vi "Report_Body.vi"(0 "report in":refnum<class "NI_report.lvclass">, 5 "Seq_Measurement":T3(array[cluster]), 7 "General_Info":T1, 9 "Log_Seq":T2(array[cluster]), 11 "error in (no error)":errorcluster) -> (6 "appended path":path, 15 "error out":errorcluster)   [LabVIEW 2023]
uses:
  <vilib>/Utility/NIReport.llb/NI_report.lvclass
  <vilib>/Utility/NIReport.llb/image depth.ctl
  <vilib>/Utility/NIReport.llb/NI_ReportGenerationCore.lvlib
panel:
  out "FFT":cluster{"f0":dbl, "df":dbl, "magnitude":dbl[]}(graph)
  out "Timesignal":waveform(dbl)(graph)
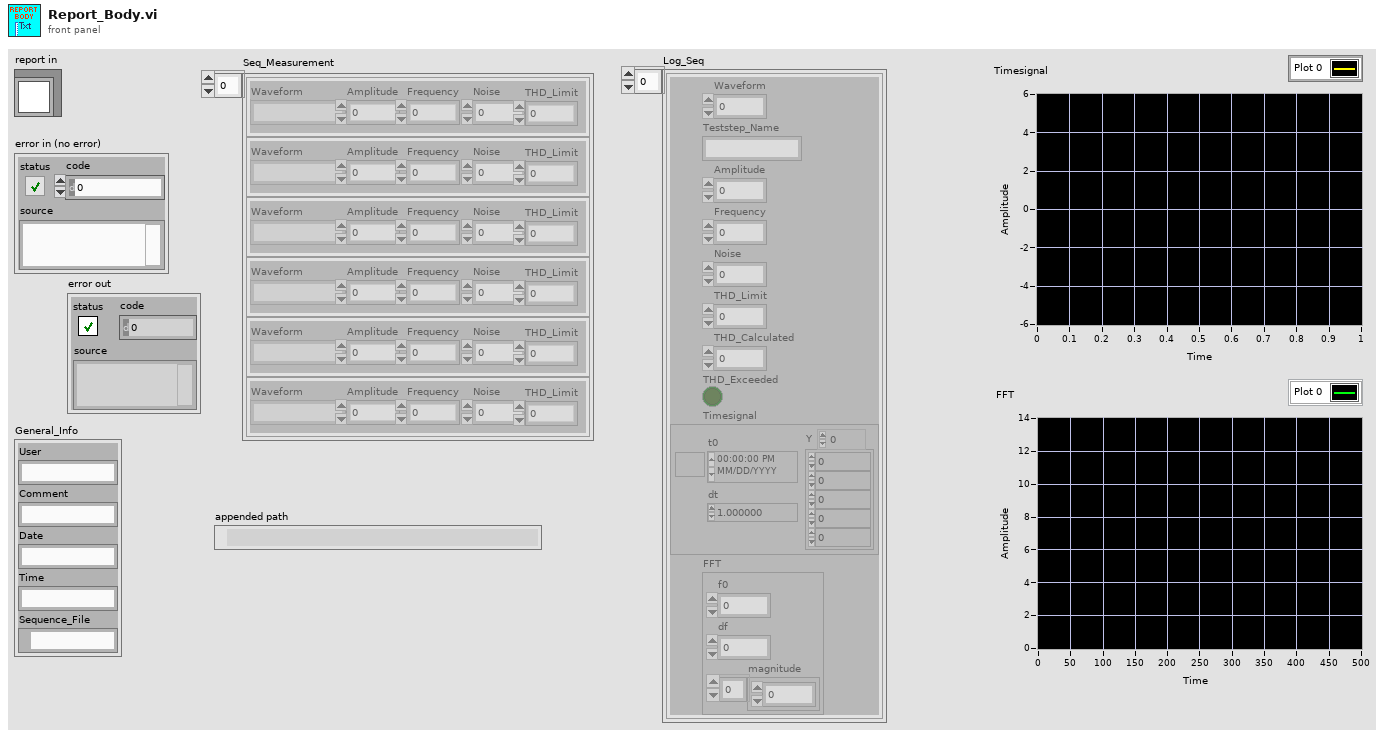
[diagram p1: front panel]
types:
  T1 = cluster{"User":string, "Comment":string, "Date":string, "Time":string, "Sequence_File":path}
  T2 = cluster{"Waveform":i32, "Teststep_Name":string, "Amplitude":dbl, "Frequency":dbl, "Noise":dbl, "THD_Limit":dbl, "THD_Calculated":dbl, "THD_Exceeded":bool, "Timesignal":waveform(dbl), "FFT":cluster{"f0":dbl, "df":dbl, "magnitude":dbl[]}}[]
  T3 = cluster{"Waveform":enum16{"", "Sine Wave", "Triangle Wave", "Square Wave", "Sawtooth Wave"}, "Amplitude":dbl, "Frequency":dbl, "Noise":dbl, "THD_Limit":dbl, "Teststep_Name":string}[]
  T4 = enum16{"open", "replace", "create", "open or create", "replace or create", "replace or create with confirmation"}
  T5 = typedef "NI_ReportGenerationCore.lvlib/image depth.ctl" = u16
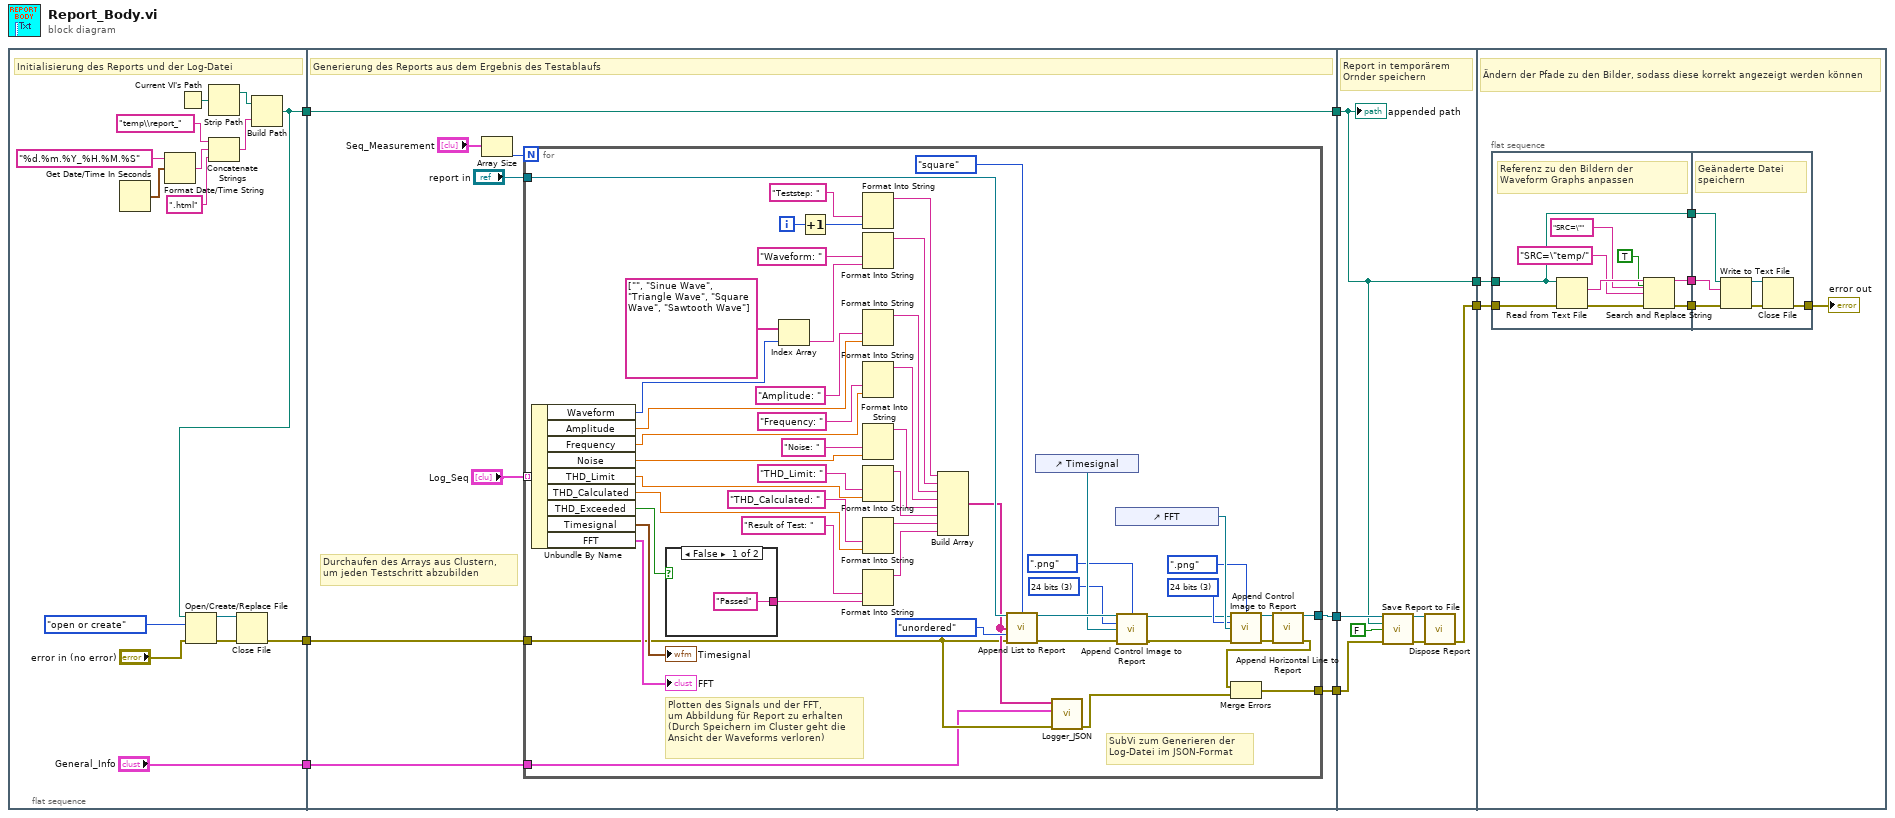
[diagram p0: block diagram]
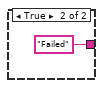
[diagram p2: hidden frame]
diagram:
  n1 = flat-sequence {
    tunnel: [w18] -> w8
    tunnel: [w10] -> w5
    tunnel: ["General_Info"] -> w3
    tunnel: w8 -> [w28]
    tunnel: [w28] -> w7
    tunnel: [w27] -> w6
    tunnel: w5 -> [w26]
    tunnel: [w25] -> w4
    tunnel: w3 -> [w24]
    tunnel: w7 -> [w89]
    tunnel: w6 -> [w93]
    tunnel: w4 -> [w92]
    tunnel: [w89] -> w2
    tunnel: [w88] -> w1
    tunnel: w2 -> [w99]
    tunnel: w1 -> [w98]
    frame #0 {
      # "Initialisierung des Reports und der Log-Datei"
      n2 = Get Date/Time In Seconds() -> (seconds since 1Jan1904=w17:timestamp)
      n3 = Format Date/Time String(time format string (%c)="%d.%m.%Y_%H.%M.%S", seconds (now)=w17) -> (date/time string=w14:string)  [unwired: 1 in]
      n4 = Current VI's Path() -> (path=w20:path)
      n5 = Strip Path(path=w20) -> (stripped path=w19:path)  [unwired: 1 out]
      n6 = Concatenate Strings("temp\\report_", w14, ".html" ("string")) -> (w12:string)
      n7 = Build Path(base path=w19, name or relative path=w12) -> (appended path=w18:path)
      n8 = Open/Create/Replace File(file path (use dialog)=w18, error in="error in (no error)", operation (0:open)=T4."open or create") -> (refnum out=w21:refnum<file>, error out=w22:errorcluster)  [unwired: 3 in, 1 out]
      n9 = Close File(refnum=w21, error in=w22) -> (error out=w10:errorcluster)  [unwired: 1 out]
    }
    frame #1 {
      # "Durchaufen des Arrays aus Clustern, \num jeden Testschritt abzubilden"
      # "Generierung des Reports aus dem Ergebnis des Testablaufs"
      n10 = Array Size(array="Seq_Measurement") -> (size(s)=w31:i32)
      n11 = for {
        N: w31 -> [_]
        tunnel: "report in" -> [w65]
        tunnel: w26 -> [w44]
        tunnel: "Log_Seq" -> [w58] mode=indexing
        tunnel: [w51] -> w27
        tunnel: [w41] -> w25
        tunnel: w24 -> [w40]
        i -> [w53]
        w33 = T5 3 items=["B&W", "4 bits", "8 bits", "24 bits"] ("image depth")
        w48 = T5 3 items=["B&W", "4 bits", "8 bits", "24 bits"] ("image depth")
        # "SubVi zum Generieren der \nLog-Datei im JSON-Format"
        # "Plotten des Signals und der FFT,\num Abbildung für Report zu erhalten\n(Durch Speichern im Cluster geht die\nAnsicht der Waveforms verloren)"
        n12 = Unbundle By Name(w58) -> ("Waveform"=w64:i32, "Amplitude"=w63:dbl, "Frequency"=w62:dbl, "Noise"=w61:dbl, "THD_Limit"=w60:dbl, "THD_Calculated"=w59:dbl, "THD_Exceeded"=w55:bool, "Timesignal"=→"Timesignal":waveform(dbl), "FFT"=→"FFT":cluster{"f0":dbl, "df":dbl, "magnitude":dbl[]})
        n13 = case shown="False" w55 {
          tunnel: ["Passed" "Failed"] -> w54
          frame False {
          }
          frame True {
          }
        }
        n14 = Index Array(array=string[] ["", "Sinue Wave", "Triangle Wave", "Square Wave", "Sawtooth Wave"], index=w64) -> (element=w81:string)
        n15 = Increment(x=w53) -> (x+1=w52:i32)
        n16 = Format Into String("Teststep: ", w52) -> (resulting string=w75:string)  [unwired: 3 in, 1 out]
        n17 = Format Into String("Waveform: ", w81) -> (resulting string=w74:string)  [unwired: 3 in, 1 out]
        n18 = Format Into String("Amplitude: ", w63) -> (resulting string=w73:string)  [unwired: 3 in, 1 out]
        n19 = Format Into String("Frequency: ", w62) -> (resulting string=w72:string)  [unwired: 3 in, 1 out]
        n20 = Format Into String("Noise: ", w61) -> (resulting string=w71:string)  [unwired: 3 in, 1 out]
        n21 = Format Into String("THD_Limit: ", w60) -> (resulting string=w70:string)  [unwired: 3 in, 1 out]
        n22 = Format Into String("THD_Calculated: ", w59) -> (resulting string=w69:string)  [unwired: 3 in, 1 out]
        n23 = Format Into String("Result of Test: ", w54) -> (resulting string=w68:string)  [unwired: 3 in, 1 out]
        n24 = Build Array(w75, w74, w73, w72, w71, w70, w69, w68) -> (w45:string[])
        n25 = call-dynamic "Append List to Report.vi"("report in"=w65, "unordered item type (default)"=enum16{"(default)", "disc", "square", "circle"}."square", "list elements"=w45, "list type (ordered)"=enum16{"unordered", "ordered"}."unordered", "error in (no error)"=w44) -> ("report out"=w39:refnum<class "NI_report.lvclass">, "error out"=w36:errorcluster)  [unwired: 7 in, 2 out]
        n26 = control-ref of="Timesignal"() -> (w35:refnum<vi>)
        n27 = call "Logger_JSON.vi"("error in"=w44, "General_Info"=w40, "appended array"=w45) -> ("error out"=w43:errorcluster)  [unwired: 8 in]
        n28 = control-ref of="FFT"() -> (w50:refnum<vi>)
        n29 = call-dynamic "Append Control Image to Report.vi"("report in"=w39, "image file type (.jpg)"=enum16{".jpg", ".png"}.".png", "image depth"=w33, "ctrl reference"=w35, "error in (no error)"=w36) -> ("report out"=w38:refnum<class "NI_report.lvclass">, "error out"=w37:errorcluster)  [unwired: 7 in, 2 out]
        n30 = call-dynamic "Append Control Image to Report.vi"("report in"=w38, "image file type (.jpg)"=enum16{".jpg", ".png"}.".png", "image depth"=w48, "ctrl reference"=w50, "error in (no error)"=w37) -> ("report out"=w47:refnum<class "NI_report.lvclass">, "error out"=w46:errorcluster)  [unwired: 7 in, 2 out]
        n31 = call-dynamic "Append Horizontal Line to Report.vi"("report in"=w47, "error in (no error)"=w46) -> ("report out"=w51:refnum<class "NI_report.lvclass">, "error out"=w42:errorcluster)  [unwired: 12 in]
        n32 = Merge Errors(w42, w43) -> (w41:errorcluster)
      }
    }
    frame #2 {
      # "Report in temporärem \nOrnder speichern"
      n33 = call-dynamic "Save Report to File.vi"("report in"=w93, "report file path"=w89, "prompt to replace? (F)"=FALSE, "error in (no error)"=w92) -> ("report out"=w91:refnum<class "NI_report.lvclass">, "error out"=w90:errorcluster)  [unwired: 10 in]
      n34 = call-dynamic "Dispose Report.vi"("report in"=w91, "error in (no error)"=w90) -> ("error out"=w88:errorcluster)  [unwired: 13 in]
      "appended path" <- w89
    }
    frame #3 {
      # "Ändern der Pfade zu den Bilder, sodass diese korrekt angezeigt werden können"
      n35 = flat-sequence {
        tunnel: [w105] -> w100
        tunnel: w99 -> [w101]
        tunnel: w98 -> [w104]
        tunnel: [w102] -> w97
        tunnel: [w101] -> w96
        tunnel: w100 -> [w115]
        tunnel: w97 -> [w114]
        tunnel: w96 -> [w113]
        tunnel: [w110] -> w95
        frame #0 {
          # "Referenz zu den Bildern der \nWaveform Graphs anpassen"
          n36 = Read from Text File(file (use dialog)=w101, error in=w104) -> (text=w109:string, error out=w103:errorcluster)  [unwired: 2 in, 2 out]
          n37 = Search and Replace String(replace all?=TRUE ("replace all? (F)"), input string=w109, search string="SRC=\"", replace string="SRC=\"temp/" ("replace string (\"\")"), error in=w103) -> (result string=w105:string, error out=w102:errorcluster)  [unwired: 3 in, 2 out]
        }
        frame #1 {
          # "Geänaderte Datei \nspeichern"
          n38 = Write to Text File(file (use dialog)=w113, text=w115, error in=w114) -> (refnum out=w112:refnum<file>, error out=w111:errorcluster)  [unwired: 1 in, 1 out]
          n39 = Close File(refnum=w112, error in=w111) -> (error out=w110:errorcluster)  [unwired: 1 out]
        }
      }
      "error out" <- w95
    }
  }
